vi "Display Data.vi"(8 "error in (no error)":errorcluster, 11 "Macro in":refnum<class "Macro.lvclass">) -> (0 "error out":errorcluster, 1 "Metadata":string, 2 "Macro Steps":string[][](array[string]), 3 "Macro out":refnum<class "Macro.lvclass">)   [LabVIEW 2020, in "MacroAssert.lvlib" / "Macro.lvclass"]
uses:
  Macro.lvclass
  Macro.lvclass/Macro.ctl
  Step/Step.lvclass
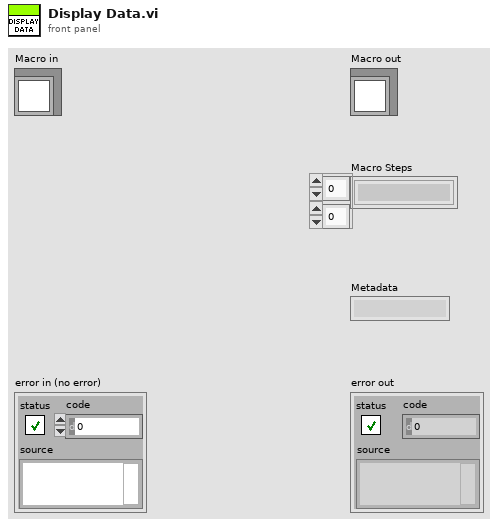
[diagram p1: front panel]
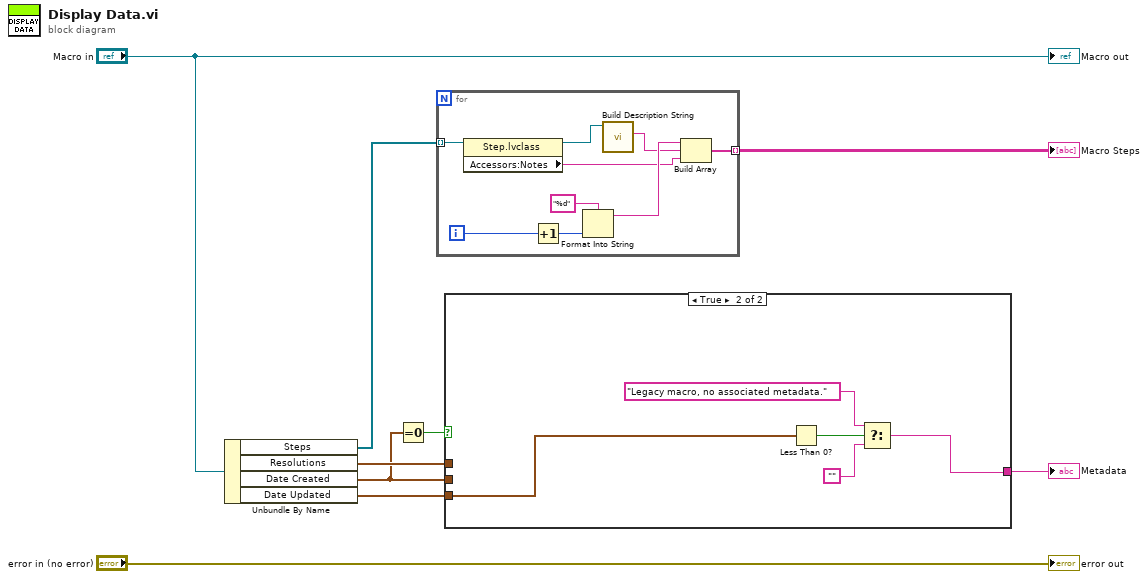
[diagram p0: block diagram]
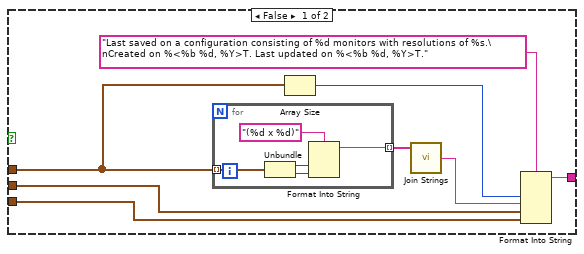
[diagram p2: hidden frame]
diagram:
  n1 = Unbundle By Name("Macro in") -> ("Steps"=w8:refnum<class "Step.lvclass">[], "Resolutions"=w6:cluster{"Width":i16, "Height":i16}[], "Date Created"=w3:timestamp, "Date Updated"=w7:timestamp)
  n2 = Equal To 0?(x=w3) -> (x = 0?=w4:bool)
  n3 = for {
    tunnel: w8 -> [w13] mode=indexing
    tunnel: [w15] -> w9 mode=indexing
    i -> [w14]
    n4 = property class="Step.lvclass"(reference=w13) -> (reference out=w11:refnum<class "Step.lvclass">, "Accessors:Notes"=w12:string)  [unwired: 1 in, 1 out]
    n5 = Increment(x=w14) -> (x+1=w18:i32)
    n6 = Format Into String(format string="%d", w18) -> (resulting string=w16:string)  [unwired: 2 in, 1 out]
    n7 = call-dynamic "Build Description String.vi"("Step in"=w11) -> ("Description"=w10:string)  [unwired: 8 in, 2 out]
    n8 = Build Array(w16, w10, w12) -> (w15:string[])
  }
  "Macro Steps" <- w9
  n9 = case shown="True" w4 {
    tunnel: w7 -> [w25 w36]
    tunnel: w3 -> [w24 _]
    tunnel: w6 -> [w22 _]
    tunnel: [w19 w32] -> w5
    frame False {
      n10 = for {
        tunnel: w22 -> [w30] mode=indexing
        tunnel: [w27] -> w21 mode=indexing
        n11 = Unbundle(w30) -> ("Width"=w28:i16, "Height"=w29:i16)
        n12 = Format Into String(format string="(%d x %d)", w28, w29) -> (resulting string=w27:string)  [unwired: 2 in, 1 out]
      }
      n13 = Array Size(array=w22) -> (size(s)=w23:i32)
      n14 = call <vilib>:"Join Strings.vi"("Strings In"=w21) -> ("String"=w20:string)  [unwired: 2 in]
      n15 = Format Into String(format string="Last saved on a configuration consisting of %d monitors with resolutions of %s.\nCreated on %<%b %d, %Y>T. Last updated on %<%b %d, %Y>T.", w23, w20, w24, w25) -> (resulting string=w19:string)  [unwired: 2 in, 1 out]
    }
    frame True {
      n16 = Less Than 0?(x=w36) -> (x < 0?=w35:bool)
      n17 = Select(t="Legacy macro, no associated metadata.", s=w35, f="") -> (s? t:f=w32:string)
    }
  }
  "Metadata" <- w5
  "error out" <- "error in (no error)"
  "Macro out" <- "Macro in"
